vi "convert_then_upload.vi"() -> ()   [LabVIEW 2016]
uses:
  subvi/Data.S3/Data.S3.lvclass
  <userlib>/_OpenG.lib/file/file.llb/File Exists - Scalar__ogtk.vi
  <userlib>/_OpenG.lib/file/file.llb/Build Path - File Names Array__ogtk.vi
panel:
  in  "POPULATE TDMS LIST":bool
  in  "folder with tdms":path
  out "Converting Indicator":bool
  in  "auto upload":bool
  out "of":i32
  out "file #":i32
  out "currently uploading file:":path
  out "errorish":string
  in  "path to aws credentials":path=path "C:/Users/phil/.aws/credentials"
  in  "aws bucket":string="levylab-data"
  out "Uploading Indicator":bool
  out "S3 upload (ms)":u32
  out "generated tdms files (w/ metadata)":path[](array[path])
  in  "UPLOAD CONVERTED":bool
  out "not itx folder":bool[](array[boolean])
  in  "e.g. SA03008N.20190801":path=path "C:/bigdata/PPMS2/SA03008N.20190801"
  in  "Tree":string[](tree)
  in  "CONVERT SELECTED":bool
  in  "OK":bool
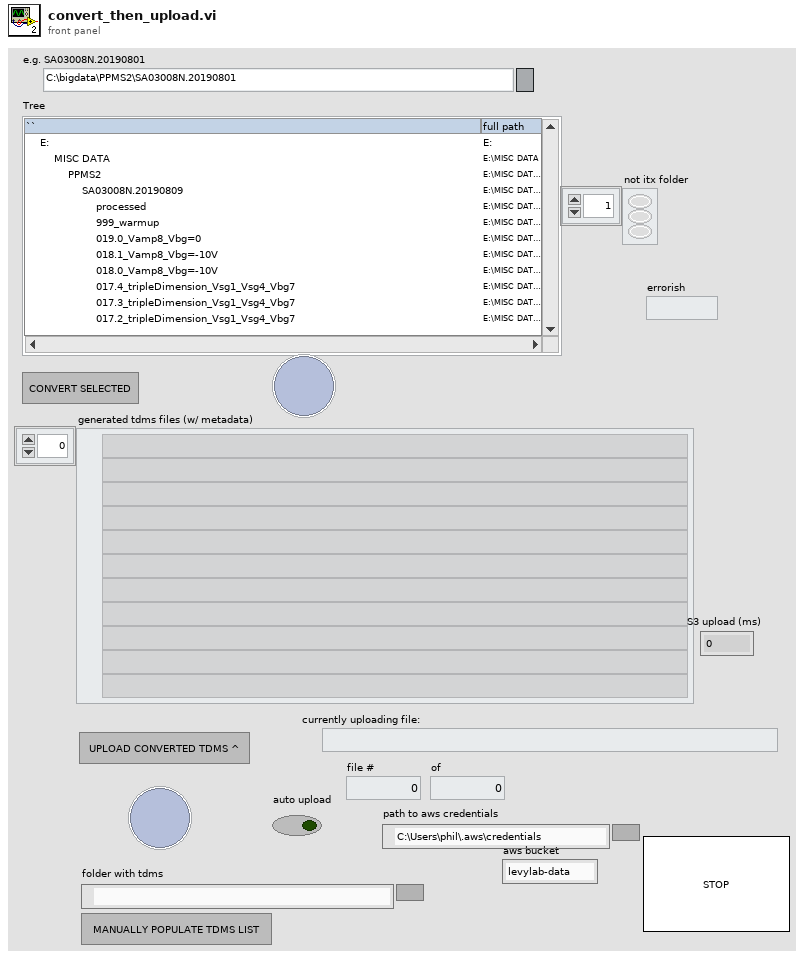
[diagram p1: front panel]
types:
  T1 = enum32{"Invalid", "Standard", "Closed", "Hidden", "Minimized", "Maximized"}
  T2 = enum32{"invalid app kind", "Development System", "Run Time System", "Student Edition", "Embedded LabVIEW", "Evaluation", "Custom"}
  T3 = cluster{"Core":cluster{"Current VI Reference":refnum<vi>, "Close Panel on Exit?":bool}, "Your Boolean data":bool, "e.g. SA03008N.20190801":path, "all expt folders (for tree)":path[], "generated tdms files":path[], "selected folders to convert":path[], "Tree":refnum<vi>, "Data.S3":refnum<class "Data.S3.lvclass">}
  T4 = cluster{"Current VI Reference":refnum<vi>, "Close Panel on Exit?":bool}
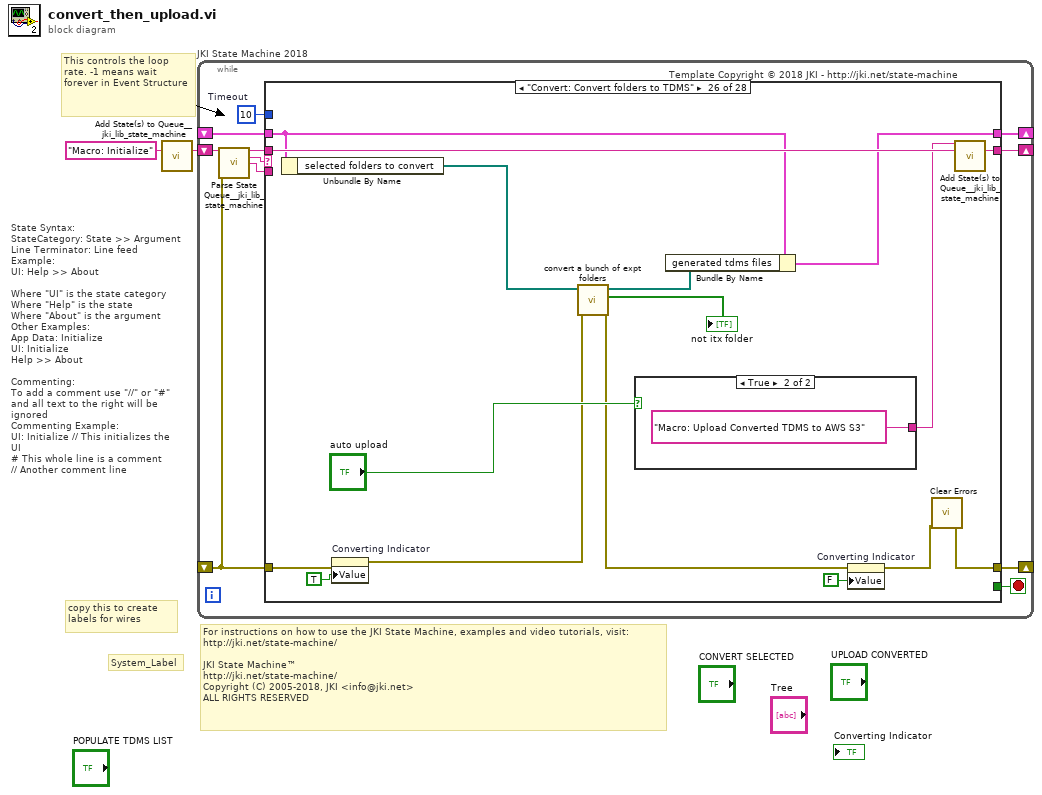
[diagram p0: block diagram]
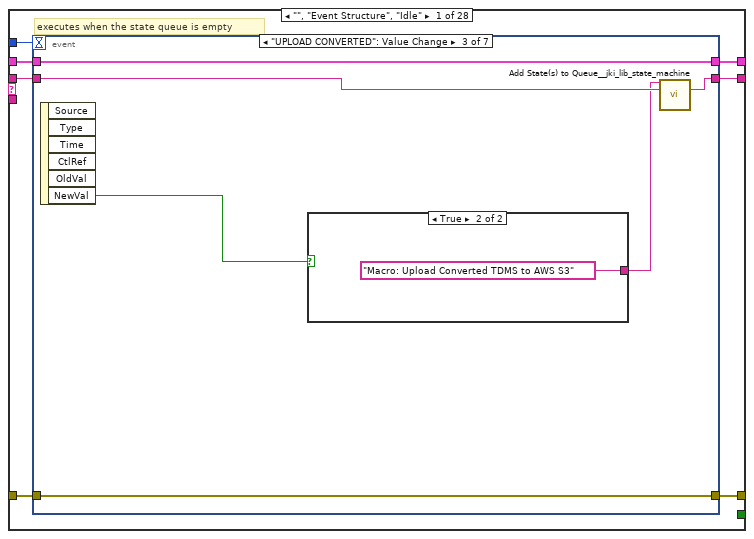
[diagram p2: hidden frame]
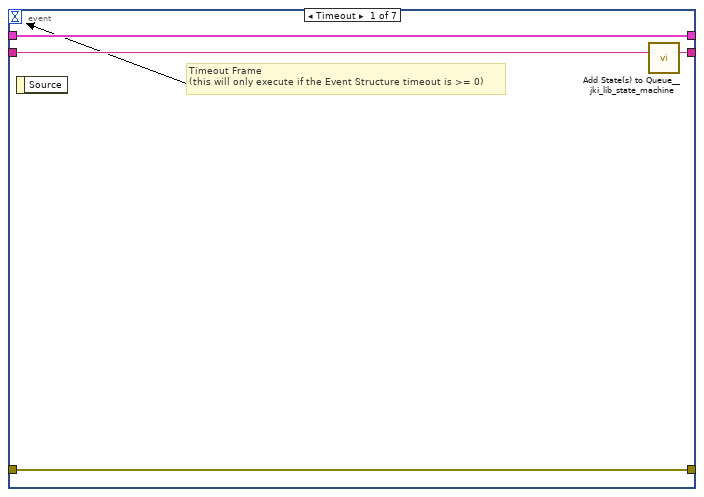
[diagram p3: hidden frame]
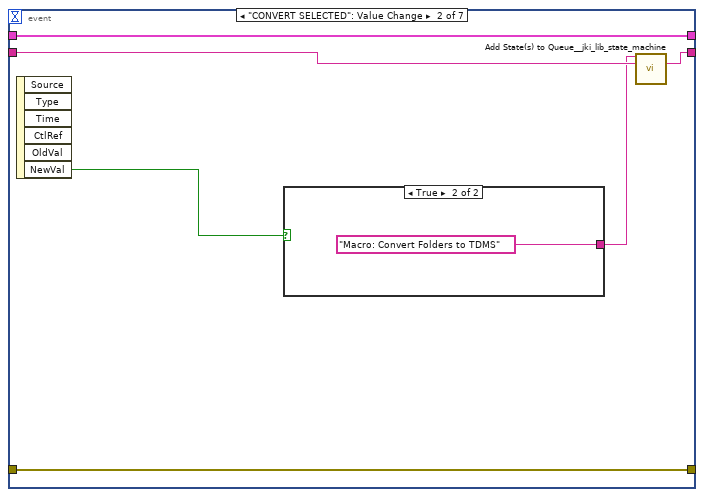
[diagram p4: hidden frame]
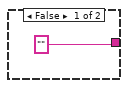
[diagram p5: hidden frame]
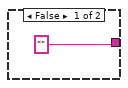
[diagram p6: hidden frame]
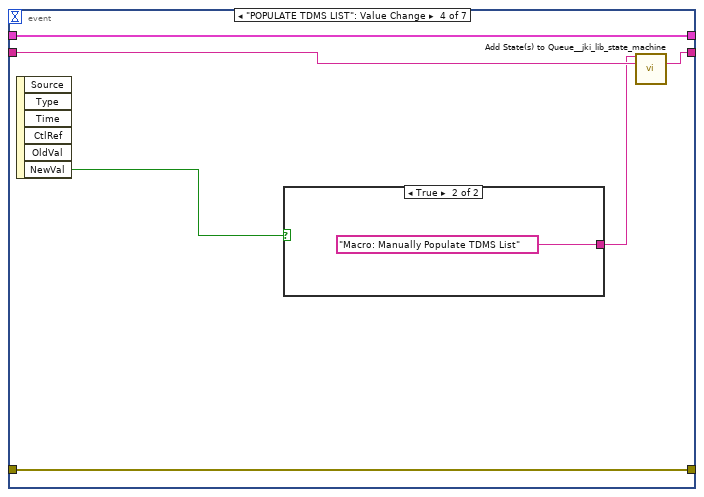
[diagram p7: hidden frame]
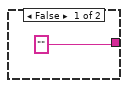
[diagram p8: hidden frame]
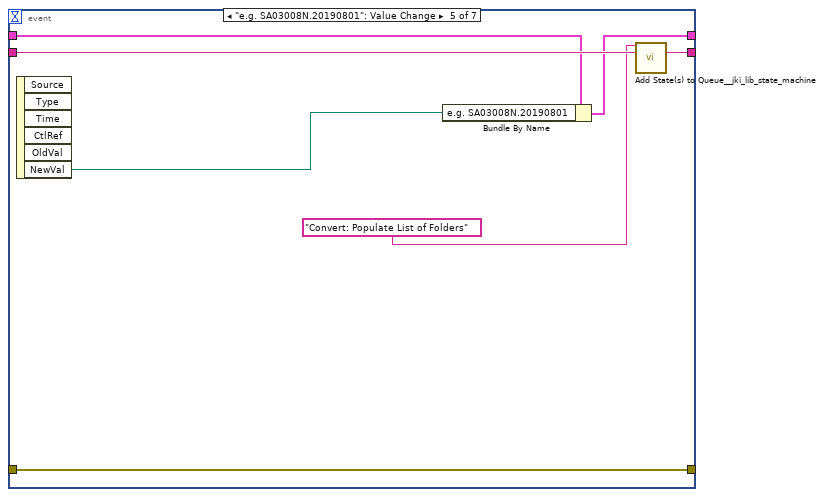
[diagram p9: hidden frame]
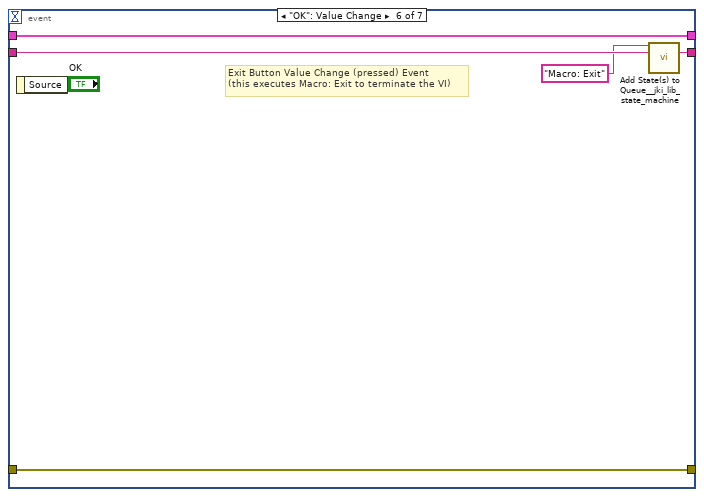
[diagram p10: hidden frame]
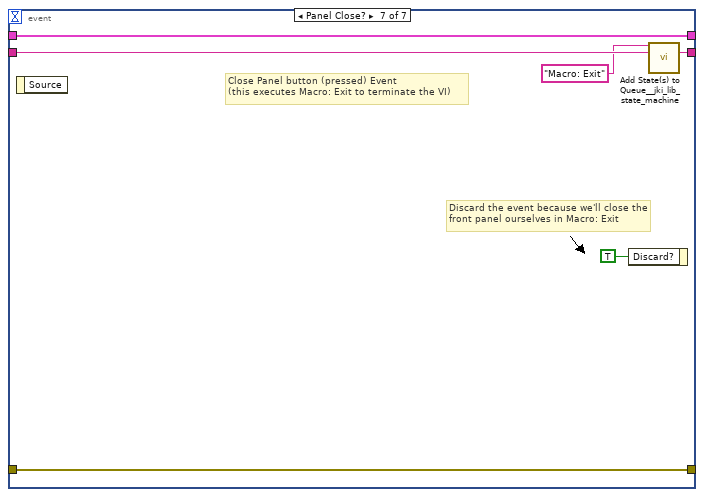
[diagram p11: hidden frame]
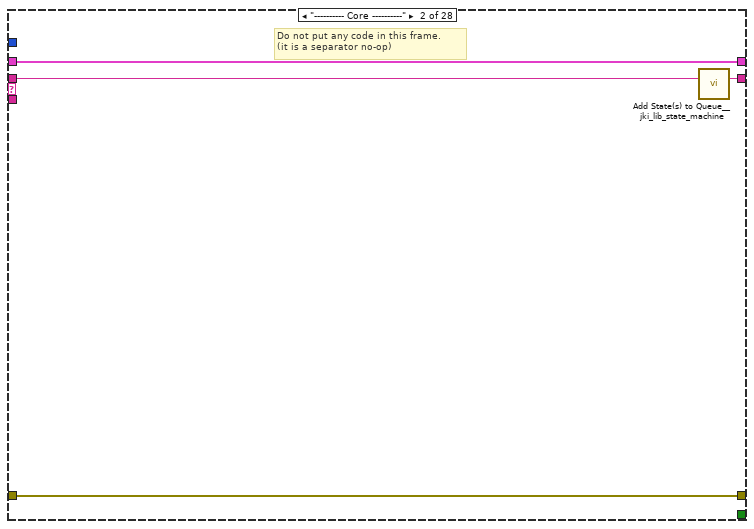
[diagram p12: hidden frame]
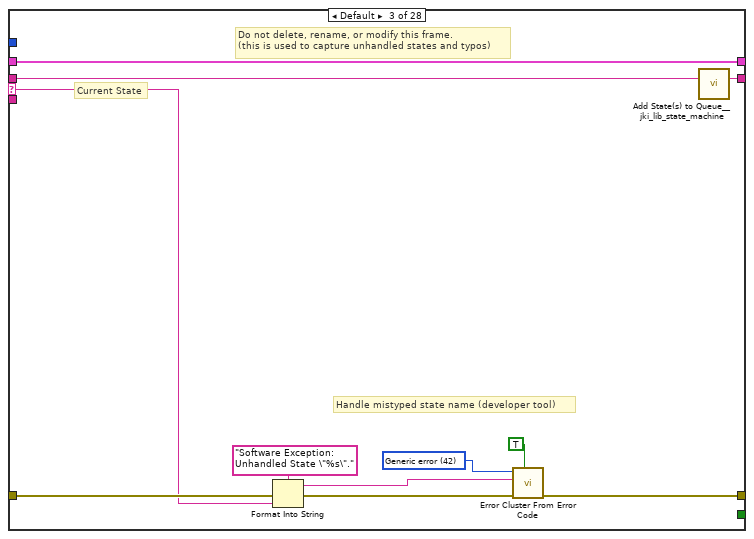
[diagram p13: hidden frame]
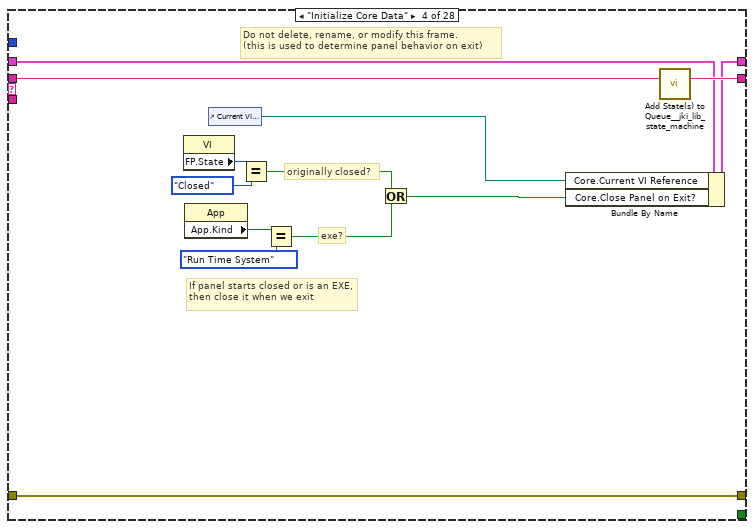
[diagram p14: hidden frame]
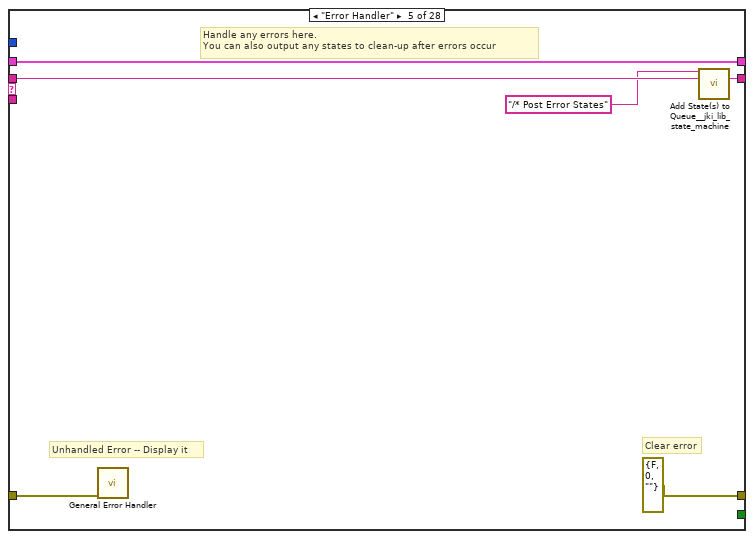
[diagram p15: hidden frame]
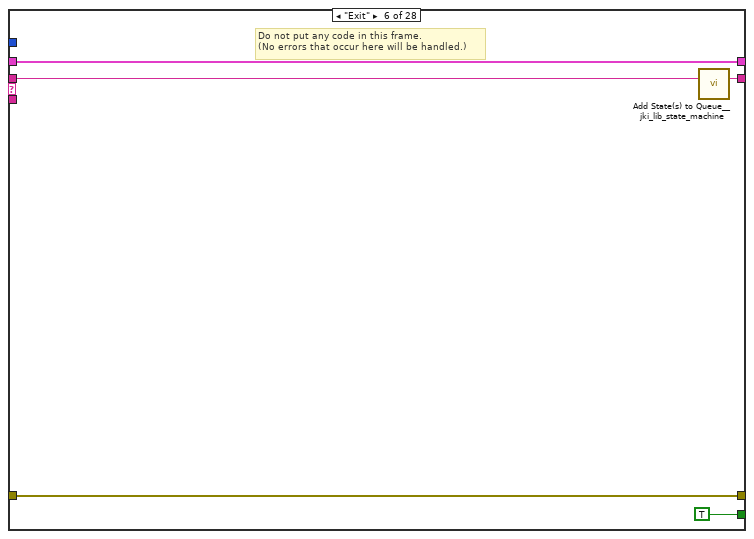
[diagram p16: hidden frame]
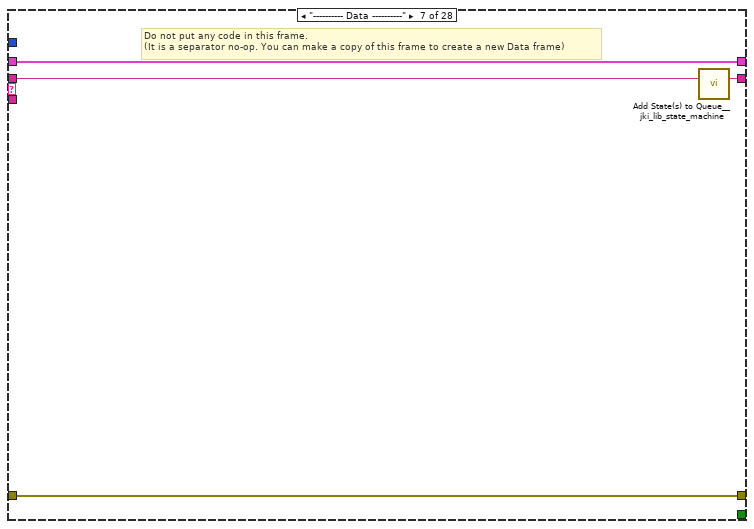
[diagram p17: hidden frame]
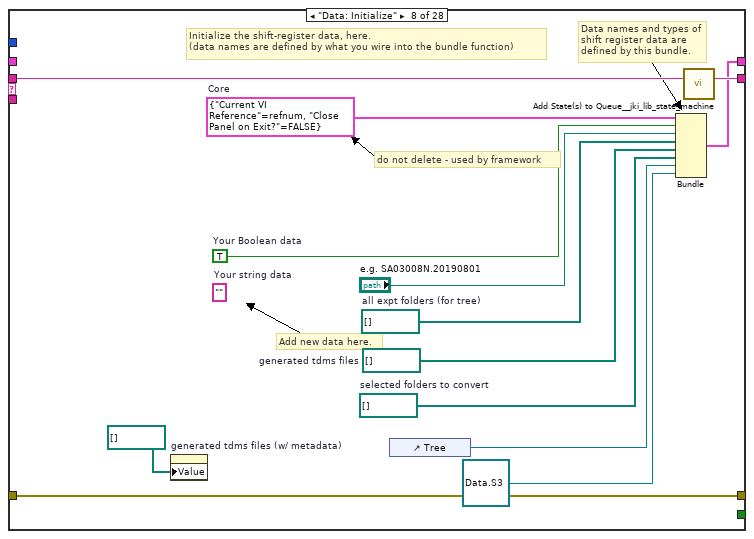
[diagram p18: hidden frame]
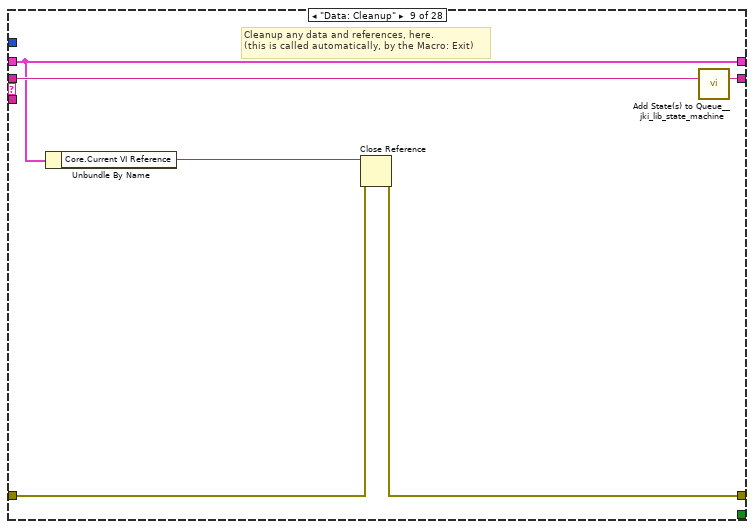
[diagram p19: hidden frame]
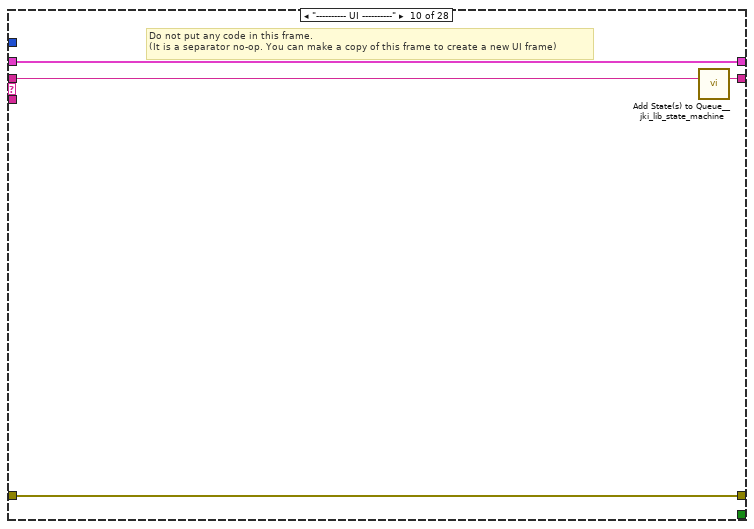
[diagram p20: hidden frame]
diagram:
  # "For instructions on how to use the JKI State Machine, examples and video tutorials, visit:\nhttp://jki.net/state-machine/\n\nJKI State Machine™\nhttp://jki.net/state-machine/\nCopyright (C) 2005-2018, JKI <info@jki.net>\nALL RIGHTS RESERVED"
  # "State Syntax:\nStateCategory: State >> Argument\nLine Terminator: Line feed\nExample:\nUI: Help >> About\n\nWhere \"UI\" is the state category\nWhere \"Help\" is the state\nWhere \"About\" is the argument\nOther Examples:\nApp Data: Initialize\nUI: Initialize\nHelp >> About\n\nCommenting:\nTo add a comment use \"//\" or \"#\" and all text to the right will be ignored\nCommenting Example:\nUI: Initialize // This initializes the UI\n# This whole line is a comment\n// Another comment line"
  # "copy this to create labels for wires"
  # "This controls the loop rate. -1 means wait forever in Event Structure"
  # "System_Label"
  n1 = call <vilib>:"Add State(s) to Queue__jki_lib_state_machine.vi"("State(s) in (\"\")"="Macro: Initialize") -> ("States Out"=w2:string)  [unwired: 14 in]
  n2 = while "JKI State Machine 2018" {
    shift-right: [w6] -> _
    shift-left: _ -> [w5]
    shift-right: [w9] -> _
    shift-left: _ -> [w3]
    shift-right: [w8] -> _
    shift-left: w2 -> [w10]
    stop <- w7 stop-if-true
    w4 = 10  # Timeout
    # "Template Copyright © 2018 JKI - http://jki.net/state-machine"
    n3 = call <vilib>:"Parse State Queue__jki_lib_state_machine.vi"("State Queue"=w10, "Error In (no error)"=w3) -> ("Remaining States"=w12:string, "Current State"=w13:string, "Arguments"=w11:string)  [unwired: 11 in]
    n4 = case shown="\"Convert: Convert folders to TDMS\"" w13 {
      selector: w13 -> [_ _ w71 _ _ _ _ _ _ _ _ _ _ _ _ _ _ _ _ _ _ _ _ _ _ _ _ _]
      tunnel: w12 -> [w20 w70 w75 w94 w100 w105 w109 w122 w128 w132 w136 w142 w153 w222 w227 w232 w237 w242 w252 w256 w275 w323 w331 w345 w359 w375 w382 w391]
      tunnel: w11 -> [_ _ _ _ _ _ _ _ _ _ _ w137 w147 _ _ _ _ _ _ _ _ _ _ _ _ _ _ _]
      tunnel: w5 -> [w18 w67 w73 w87 w97 w103 w106 _ w123 w129 w134 w140 w149 w219 w224 w229 w234 w239 w249 w253 w259 w316 w328 w339 w356 w371 w379 w386]
      tunnel: [w17 w68 w77 w91 errorcluster {"status"=FALSE, "code"=0, "source"=""} ("error out") w102 w107 w119 w124 w130 w133 w138 w150 w220 w225 w230 w235 w240 w250 w254 w273 w313 w329 w332 w351 w360 w380 w388] -> w9
      tunnel: w3 -> [w16 w68 w76 w91 w96 w102 w107 w119 w125 w130 w133 w139 w151 w220 w225 w230 w235 w240 w250 w254 w273 w312 w329 w335 w352 w366 w380 w389]
      tunnel: [w19 w69 w74 w93 w99 w104 w108 w121 w127 w131 w135 w141 w152 w221 w226 w231 w236 w241 w251 w255 w274 w322 w330 w344 w358 w374 w381 w390] -> w8
      tunnel: [_ _ _ _ _ TRUE _ _ _ _ _ _ _ _ _ _ _ _ _ _ _ _ _ _ _ _ _ _] -> w7
      tunnel: [w15 w67 w73 w92 w97 w103 w106 w120 w123 w129 w134 w140 w149 w219 w224 w229 w234 w239 w249 w253 w258 w315 w328 w343 w357 w370 w379 w385] -> w6
      tunnel: w4 -> [w14 _ _ _ _ _ _ _ _ _ _ _ _ _ _ _ _ _ _ _ _ _ _ _ _ _ _ _]
      frame "", "Event Structure", "Idle" {
        # "executes when the state queue is empty"
        n5 = event shown="[2] \"UPLOAD CONVERTED\": Value Change" {
          selector: _ -> [_ _ _ _ _ _ _]
          dyn-events: _ -> [_ _ _ _ _ _ _]
          timeout: w14 -> [_ _ _ _ _ _ _]
          tunnel: w20 -> [w24 w28 w36 w44 w54 w60 w66]
          tunnel: [w23 w29 w37 w45 w55 w59 w65] -> w19
          tunnel: w18 -> [w21 w30 w38 w46 w51 w57 w63]
          tunnel: [w22 w27 w35 w43 w53 w58 w64] -> w17
          tunnel: w16 -> [w22 w27 w35 w43 w53 w58 w64]
          tunnel: [w21 w30 w38 w46 w50 w57 w63] -> w15
          event Timeout {
            # "Timeout Frame\n(this will only execute if the Event Structure timeout is >= 0)"
            n6 = event-data() -> ()  [unwired: 1 in, 1 out]
            n7 = call <vilib>:"Add State(s) to Queue__jki_lib_state_machine.vi"("State(s) in (\"\")"=w24) -> ("States Out"=w23:string)  [unwired: 14 in]
          }
          event "CONVERT SELECTED": Value Change {
            n8 = event-data() -> ("NewVal"=w26:bool)  [unwired: 1 in, 5 out]
            n9 = case shown="True" w26 {
              tunnel: ["" "Macro: Convert Folders to TDMS"] -> w25
              frame False {
              }
              frame True {
              }
            }
            n10 = call <vilib>:"Add State(s) to Queue__jki_lib_state_machine.vi"("State(s) in Front (\"\")"=w25, "State(s) in (\"\")"=w28) -> ("States Out"=w29:string)  [unwired: 13 in]
          }
          event "UPLOAD CONVERTED": Value Change {
            n11 = event-data() -> ("NewVal"=w34:bool)  [unwired: 1 in, 5 out]
            n12 = case shown="True" w34 {
              tunnel: ["" "Macro: Upload Converted TDMS to AWS S3"] -> w33
              frame False {
              }
              frame True {
              }
            }
            n13 = call <vilib>:"Add State(s) to Queue__jki_lib_state_machine.vi"("State(s) in Front (\"\")"=w33, "State(s) in (\"\")"=w36) -> ("States Out"=w37:string)  [unwired: 13 in]
          }
          event "POPULATE TDMS LIST": Value Change {
            n14 = event-data() -> ("NewVal"=w42:bool)  [unwired: 1 in, 5 out]
            n15 = case shown="True" w42 {
              tunnel: ["" "Macro: Manually Populate TDMS List"] -> w41
              frame False {
              }
              frame True {
              }
            }
            n16 = call <vilib>:"Add State(s) to Queue__jki_lib_state_machine.vi"("State(s) in Front (\"\")"=w41, "State(s) in (\"\")"=w44) -> ("States Out"=w45:string)  [unwired: 13 in]
          }
          event "e.g. SA03008N.20190801": Value Change {
            n17 = event-data() -> ("NewVal"=w49:path)  [unwired: 1 in, 5 out]
            n18 = Bundle By Name(cluster=w51, "e.g. SA03008N.20190801"=w49) -> (w50:T3)
            n19 = call <vilib>:"Add State(s) to Queue__jki_lib_state_machine.vi"("State(s) in Front (\"\")"="Convert: Populate List of Folders", "State(s) in (\"\")"=w54) -> ("States Out"=w55:string)  [unwired: 13 in]
          }
          event "OK": Value Change {
            # "Exit Button Value Change (pressed) Event\n(this executes Macro: Exit to terminate the VI)"
            n20 = event-data() -> ()  [unwired: 1 in, 1 out]
            n21 = call <vilib>:"Add State(s) to Queue__jki_lib_state_machine.vi"("State(s) in Front (\"\")"="Macro: Exit", "State(s) in (\"\")"=w60) -> ("States Out"=w59:string)  [unwired: 13 in]
          }
          event Panel Close? {
            # "Discard the event because we'll close the front panel ourselves in Macro: Exit"
            # "Close Panel button (pressed) Event\n(this executes Macro: Exit to terminate the VI)"
            n22 = event-data() -> ()  [unwired: 1 in, 1 out]
            n23 = event-data("Discard?"=TRUE) -> ()  [unwired: 1 in, 1 out]
            n24 = call <vilib>:"Add State(s) to Queue__jki_lib_state_machine.vi"("State(s) in Front (\"\")"="Macro: Exit", "State(s) in (\"\")"=w66) -> ("States Out"=w65:string)  [unwired: 13 in]
          }
        }
      }
      frame "---------- Core ----------" {
        # "Do not put any code in this frame.\n(it is a separator no-op)"
        n25 = call <vilib>:"Add State(s) to Queue__jki_lib_state_machine.vi"("State(s) in (\"\")"=w70) -> ("States Out"=w69:string)  [unwired: 14 in]
      }
      frame Default {
        w80 = 42 items=["No error", "Argument error", "Memory is full", "Out of zone", "End of file", "File already open", "Generic file I/O error", "File not found", "File permission error", "Disk is full", "Duplicate path", "Too many files open", "System feature not enabled", "Resource file not found", "Cannot add resource", "Resource not found", "Image not found", "Image memory error", "Pen does not exist", "Config type invalid", "Config token not found", "Config parse error", "Config memory error", "Bad external code format", "Bad external code offset", "External code not present", "Null window", "Destroy window error", "Null menu", "Print aborted", "Bad print record", "Print driver error", "Windows error during printing", "Memory error during printing", "Print dialog error", "Generic print error", "Invalid device refnum", "Device not found", "Device parameter error", "Device unit error", "Cannot open device", "Device call aborted", "Generic error", "Cancelled by user", "Object ID too low", "Object ID too high", "Object not in heap", "Unknown heap", "Unknown object (invalid DefProc)", "Unknown object (DefProc not in table)", "Message out of range", "Invalid (null) method", "Unknown message", "Manager call not supported", "Bad address", "Network operation in progress", "Network operation timed out", "Connection is busy", "Network attribute not supported", "Network error", "Address in use", "System out of memory", "Connection aborted", "Connection refused", "Not connected", "Already connected", "Connection closed", "Initialization error (interapplication manager)", "Bad occurrence", "Wait on unbound occurrence handler", "Occurrence queue overflow", "Datalog type conflict", "Unused", "Unrecognized type (interapplication manager)", "Memory corrupt", "Failed to make temporary DLL", "Old CIN version", "Drag socket not found", "Failed to load drop-object", "Failed to register OLE object", "Failed to release OLE object", "Format specifier type mismatch", "Unknown format specifier", "Too few format specifiers", "Too many format specifiers", "Scan failed", "Newer CIN version", "Error converting to variant", "Runtime menu error", "Password tampered", "Variant attribute not found", "Incompatible variant data type", "Event data is not available", "Event Store is not present", "Occurrence is not found", "Event Queue is not created", "Event info is not available", "Refnum passed is NULL", "Error retrieving Class GUID", "Error retrieving CoClass GUID", "Error retrieving TypeLib GUID.", "Bad built application magic bytes.", "Specific driver is different from the specific driver associated with the Logical Name.", "There is no session opened to the class driver.", "Max Error", "MAX - Error with config objects", "MAX - Error loading configuration", "MAX - Group not supported"]
        # "Current State"
        # "Do not delete, rename, or modify this frame.\n(this is used to capture unhandled states and typos)"
        # "Handle mistyped state name (developer tool)"
        n26 = Format Into String(format string="Software Exception: Unhandled State \"%s\"." ("message"), error in=w76, w71) -> (resulting string=w79:string, error out=w78:errorcluster)  [unwired: 1 in]
        n27 = call <vilib>:"Error Cluster From Error Code.vi"("show call chain? (False)"=TRUE, "error in (no error)"=w78, "error message (\"\")"=w79, "error code (0)"=w80) -> ("error out"=w77:errorcluster)  [unwired: 5 in]
        n28 = call <vilib>:"Add State(s) to Queue__jki_lib_state_machine.vi"("State(s) in (\"\")"=w75) -> ("States Out"=w74:string)  [unwired: 14 in]
      }
      frame "Initialize Core Data" {
        # "Do not delete, rename, or modify this frame.\n(this is used to determine panel behavior on exit)"
        # "originally closed?"
        # "exe?"
        # "If panel starts closed or is an EXE, then close it when we exit"
        n29 = property class="VI"() -> ("FP.State"=w84:T1)  [unwired: 2 in, 2 out]
        n30 = property class="App"() -> ("App.Kind"=w90:T2)  [unwired: 2 in, 2 out]
        n31 = control-ref of="Current VI Reference"() -> (w85:refnum<vi>)
        n32 = Equal?(x=w84, y=T1."Closed" ("Front Panel Window:State")) -> (x = y?=w82:bool)
        n33 = Equal?(x=w90, y=T2."Run Time System" ("Application:Kind")) -> (x = y?=w88:bool)
        n34 = Or(x=w82, y=w88) -> (x .or. y?=w86:bool)
        n35 = Bundle By Name(cluster=w87, "Core.Current VI Reference"=w85, "Core.Close Panel on Exit?"=w86) -> (w92:T3)
        n36 = call <vilib>:"Add State(s) to Queue__jki_lib_state_machine.vi"("State(s) in (\"\")"=w94) -> ("States Out"=w93:string)  [unwired: 14 in]
      }
      frame "Error Handler" {
        # "Unhandled Error -- Display it"
        # "Handle any errors here.\nYou can also output any states to clean-up after errors occur"
        # "Clear error"
        n37 = call <vilib>:"General Error Handler.vi"("error in (no error)"=w96) -> ()  [unwired: 10 in, 5 out]
        n38 = call <vilib>:"Add State(s) to Queue__jki_lib_state_machine.vi"("State(s) in Front (\"\")"="/* Post Error States", "State(s) in (\"\")"=w100) -> ("States Out"=w99:string)  [unwired: 13 in]
      }
      frame "Exit" {
        # "Do not put any code in this frame.\n(No errors that occur here will be handled.)"
        n39 = call <vilib>:"Add State(s) to Queue__jki_lib_state_machine.vi"("State(s) in (\"\")"=w105) -> ("States Out"=w104:string)  [unwired: 14 in]
      }
      frame "---------- Data ----------" {
        # "Do not put any code in this frame.\n(It is a separator no-op. You can make a copy of this frame to create a new Data frame)"
        n40 = call <vilib>:"Add State(s) to Queue__jki_lib_state_machine.vi"("State(s) in (\"\")"=w109) -> ("States Out"=w108:string)  [unwired: 14 in]
      }
      frame "Data: Initialize" {
        w114 = path[] []  # selected folders to convert
        w115 = path[] []  # generated tdms files
        w116 = path[] []  # all expt folders (for tree)
        w117 = T4 {"Current VI Reference"=refnum, "Close Panel on Exit?"=FALSE}  # Core
        w118 = TRUE  # Your Boolean data
        (unwired) ""  # Your string data
        # "do not delete - used by framework"
        # "Add new data here."
        # "Data names and types of shift register data are defined by this bundle."
        # "Initialize the shift-register data, here.\n(data names are defined by what you wire into the bundle function)"
        n41 = property on="generated tdms files (w/ metadata)" class="Arr (strict)"("Value"=path[] [] ("converted folders")) -> ()  [unwired: 2 in, 2 out]
        n42 = control-ref of="Tree"() -> (w112:refnum<vi>)
        n43 = Bundle("Core"=w117, "Your Boolean data"=w118, "e.g. SA03008N.20190801"="e.g. SA03008N.20190801", "all expt folders (for tree)"=w116, "generated tdms files"=w115, "selected folders to convert"=w114, "Tree"=w112, "Data.S3"=refnum<class "Data.S3.lvclass"> refnum) -> (w120:T3)  [unwired: 1 in]
        n44 = call <vilib>:"Add State(s) to Queue__jki_lib_state_machine.vi"("State(s) in (\"\")"=w122) -> ("States Out"=w121:string)  [unwired: 14 in]
      }
      frame "Data: Cleanup" {
        # "Cleanup any data and references, here.\n(this is called automatically, by the Macro: Exit)"
        n45 = Unbundle By Name(w123) -> ("Core.Current VI Reference"=w126:refnum<vi>)
        n46 = Close Reference(reference=w126, error in (no error)=w125) -> (error out=w124:errorcluster)
        n47 = call <vilib>:"Add State(s) to Queue__jki_lib_state_machine.vi"("State(s) in (\"\")"=w128) -> ("States Out"=w127:string)  [unwired: 14 in]
      }
      frame "---------- UI ----------" {
        # "Do not put any code in this frame.\n(It is a separator no-op. You can make a copy of this frame to create a new UI frame)"
        n48 = call <vilib>:"Add State(s) to Queue__jki_lib_state_machine.vi"("State(s) in (\"\")"=w132) -> ("States Out"=w131:string)  [unwired: 14 in]
      }
      frame "UI: Initialize" {
        # "Initialize the User Interface, here.\n(this is called automatically, by the Macro: Init)"
        n49 = call <vilib>:"Add State(s) to Queue__jki_lib_state_machine.vi"("State(s) in (\"\")"=w136) -> ("States Out"=w135:string)  [unwired: 14 in]
      }
      frame "UI: Cursor Set" {
        # "Argument"
        # "Set and Unset Cursor Busy.\n(Usage: \"UI: Cursor Set >> Busy|Idle\")"
        n50 = case shown="\"Idle\", Default" w137 {
          tunnel: w139 -> [w144 w146]
          tunnel: [w143 w145] -> w138
          frame "Idle", Default {
            n51 = call <vilib>:"Unset Busy.vi"("error in (no error)"=w144) -> ("error out"=w143:errorcluster)  [unwired: 10 in]
          }
          frame "Busy" {
            n52 = call <vilib>:"Set Busy.vi"("error in (no error)"=w146) -> ("error out"=w145:errorcluster)  [unwired: 9 in, 1 out]
          }
        }
        n53 = call <vilib>:"Add State(s) to Queue__jki_lib_state_machine.vi"("State(s) in (\"\")"=w142) -> ("States Out"=w141:string)  [unwired: 14 in]
      }
      frame "UI: Front Panel State" {
        # "Argument"
        # "Set Front Panel Open or Closed\n(Usage: \"UI: Front Panel State >> Open|Close\")"
        n54 = Unbundle By Name(w149) -> ("Core.Current VI Reference"=w148:refnum<vi>)
        n55 = case shown="\"Minimize\", \"Minimized\"" w147 {
          tunnel: w151 -> [w159 w174 w185 w198 w211]
          tunnel: [w161 w175 w187 w200 w213] -> w150
          tunnel: w148 -> [w160 w172 w186 w199 w212]
          frame "Open", "Standard", Default {
            w154 = T1."Standard" ("State")
            n56 = property class="VI"(reference=w160, error in=w159) -> (reference out=w157:refnum<vi>, error out=w158:errorcluster, "FP.State"=w156:T1)
            n57 = Not Equal?(x=w156, y=w154) -> (x != y?=w155:bool)
            n58 = case shown="True" w155 {
              tunnel: [w165 w167] -> w161
              tunnel: w158 -> [w164 w167]
              tunnel: w157 -> [w163 _]
              tunnel: w154 -> [w162 _]
              frame True {
                n59 = invoke class="VI" method="FP.Open"(reference=w163, error in=w164, "Activate"=TRUE, "State"=w162) -> (error out=w165:errorcluster)  [unwired: 1 in, 4 out]
              }
              frame False {
              }
            }
          }
          frame "Close", "Closed" {
            n60 = property class="VI"(reference=w172, error in=w174) -> (reference out=w171:refnum<vi>, error out=w173:errorcluster, "FP.State"=w169:T1)
            n61 = Not Equal?(x=w169, y=T1."Closed" ("Front Panel Window:State")) -> (x != y?=w168:bool)
            n62 = case shown="True" w168 {
              tunnel: [w176 w179] -> w175
              tunnel: w173 -> [w176 w178]
              tunnel: w171 -> [_ w177]
              frame False {
              }
              frame True {
                n63 = invoke class="VI" method="FP.Close"(reference=w177, error in=w178) -> (error out=w179:errorcluster)  [unwired: 1 in, 2 out]
              }
            }
          }
          frame "Hidden", "Hide" {
            w180 = T1."Hidden" ("State")
            n64 = property class="VI"(reference=w186, error in=w185) -> (reference out=w183:refnum<vi>, error out=w184:errorcluster, "FP.State"=w182:T1)
            n65 = Not Equal?(x=w182, y=w180) -> (x != y?=w181:bool)
            n66 = case shown="True" w181 {
              tunnel: [w191 w192] -> w187
              tunnel: w184 -> [w190 w192]
              tunnel: w183 -> [w189 _]
              tunnel: w180 -> [w188 _]
              frame True {
                n67 = invoke class="VI" method="FP.Open"(reference=w189, error in=w190, "State"=w188) -> (error out=w191:errorcluster)  [unwired: 2 in, 4 out]
              }
              frame False {
              }
            }
          }
          frame "Minimize", "Minimized" {
            w193 = T1."Minimized" ("State")
            n68 = property class="VI"(reference=w199, error in=w198) -> (reference out=w196:refnum<vi>, error out=w197:errorcluster, "FP.State"=w195:T1)
            n69 = Not Equal?(x=w195, y=w193) -> (x != y?=w194:bool)
            n70 = case shown="True" w194 {
              tunnel: [w204 w205] -> w200
              tunnel: w197 -> [w203 w205]
              tunnel: w196 -> [w202 _]
              tunnel: w193 -> [w201 _]
              frame True {
                n71 = invoke class="VI" method="FP.Open"(reference=w202, error in=w203, "State"=w201) -> (error out=w204:errorcluster)  [unwired: 2 in, 4 out]
              }
              frame False {
              }
            }
          }
          frame "Maximize", "Maximized" {
            w206 = T1."Maximized" ("State")
            n72 = property class="VI"(reference=w212, error in=w211) -> (reference out=w209:refnum<vi>, error out=w210:errorcluster, "FP.State"=w208:T1)
            n73 = Not Equal?(x=w208, y=w206) -> (x != y?=w207:bool)
            n74 = case shown="True" w207 {
              tunnel: [w217 w218] -> w213
              tunnel: w210 -> [w216 w218]
              tunnel: w209 -> [w215 _]
              tunnel: w206 -> [w214 _]
              frame True {
                n75 = invoke class="VI" method="FP.Open"(reference=w215, error in=w216, "State"=w214) -> (error out=w217:errorcluster)  [unwired: 2 in, 4 out]
              }
              frame False {
              }
            }
          }
        }
        n76 = call <vilib>:"Add State(s) to Queue__jki_lib_state_machine.vi"("State(s) in (\"\")"=w153) -> ("States Out"=w152:string)  [unwired: 14 in]
      }
      frame "---------- Macro ----------" {
        # "Do not put any code in this frame.\n(It is a separator no-op. You can make a copy of this frame to create a new Macro frame)"
        n77 = call <vilib>:"Add State(s) to Queue__jki_lib_state_machine.vi"("State(s) in (\"\")"=w222) -> ("States Out"=w221:string)  [unwired: 14 in]
      }
      frame "Macro: Initialize" {
        w223 = "Data: Initialize\nInitialize Core Data\nUI: Initialize\nUI: Front Panel State >> Open\nConvert: Populate List of Folders\nAWS: Initialize"  # Data: Initialize Initialize Core Data UI: Initialize UI: Front Panel State >> Open Convert: Populate List of Folders AWS: Initialize
        # "Initialization Macro\n(This is called once, when the VI starts)"
        n78 = call <vilib>:"Add State(s) to Queue__jki_lib_state_machine.vi"("State(s) in Front (\"\")"=w223, "State(s) in (\"\")"=w227) -> ("States Out"=w226:string)  [unwired: 13 in]
      }
      frame "Macro: Convert Folders to TDMS" {
        # "Initialization Macro\n(This is called once, when the VI starts)"
        n79 = call <vilib>:"Add State(s) to Queue__jki_lib_state_machine.vi"("State(s) in Front (\"\")"="Convert: Obtain Selected Folders\nConvert: Convert folders to TDMS\nConvert: Update TDMS List", "State(s) in (\"\")"=w232) -> ("States Out"=w231:string)  [unwired: 13 in]
      }
      frame "Macro: Upload Converted TDMS to AWS S3" {
        # "Initialization Macro\n(This is called once, when the VI starts)"
        n80 = call <vilib>:"Add State(s) to Queue__jki_lib_state_machine.vi"("State(s) in Front (\"\")"="AWS: Upload Converted TDMS", "State(s) in (\"\")"=w237) -> ("States Out"=w236:string)  [unwired: 13 in]
      }
      frame "Macro: Manually Populate TDMS List" {
        # "Initialization Macro\n(This is called once, when the VI starts)"
        n81 = call <vilib>:"Add State(s) to Queue__jki_lib_state_machine.vi"("State(s) in Front (\"\")"="Convert: Populate TDMS List from Folder\nConvert: Update TDMS List", "State(s) in (\"\")"=w242) -> ("States Out"=w241:string)  [unwired: 13 in]
      }
      frame "Macro: Exit" {
        # "Exit Macro\n(This is called once, when the VI exits)"
        n82 = Unbundle By Name(w249) -> ("Core.Close Panel on Exit?"=w248:bool)
        n83 = Select(t="UI: Front Panel State >> Close", s=w248, f="") -> (s? t:f=w245:string)
        n84 = call <vilib>:"Add State(s) to Queue__jki_lib_state_machine.vi"("State(s) in (\"\")"=w245, "State(s) at Back (\"\")"="Data: Cleanup\nExit") -> ("States Out"=w243:string)  [unwired: 13 in]
        n85 = call <vilib>:"Add State(s) to Queue__jki_lib_state_machine.vi"("State(s) in Front (\"\")"=w243, "State(s) in (\"\")"=w252) -> ("States Out"=w251:string)  [unwired: 13 in]
      }
      frame "---------- AWS ----------" {
        # "Template Separator\n(You can make a copy of, or modify, this frame)"
        n86 = Unbundle By Name(w253) -> ()  [unwired: 1 out]
        n87 = call <vilib>:"Add State(s) to Queue__jki_lib_state_machine.vi"("State(s) in (\"\")"=w256) -> ("States Out"=w255:string)  [unwired: 14 in]
      }
      frame "AWS: Upload Converted TDMS" {
        # "Template Separator\n(You can make a copy of, or modify, this frame)"
        # "Your code here.\n(You can make a copy of, or modify, this frame)"
        n88 = control-ref of="Uploading Indicator"() -> (w269:refnum<vi>)
        n89 = property on="Property Node" class="Bool (strict)"(reference=w269, "Value"=TRUE ("Downloading Indicator")) -> (reference out=w268:refnum<vi>, error out=w267:errorcluster)  [unwired: 1 in]
        n90 = Unbundle By Name(w259) -> ("generated tdms files"=w257:path[], "Data.S3"=w272:refnum<class "Data.S3.lvclass">)
        n91 = call <userlib>:"Tick Count (ms)__ogtk.vi"("error in (no error)"=w267) -> ("error out"=w266:errorcluster, "millisecond timer value"=w262:u32)  [unwired: 9 in]
        n92 = for {
          tunnel: w272 -> [w293]
          tunnel: [w285] -> w260
          shift-right: [w278] -> w265
          shift-left: w266 -> [w286]
          tunnel: w257 -> [w283] mode=indexing
          tunnel: w257 -> [w280]
          i -> [w282]
          w288 = "/"
          # "PPMS2"
          # "reformat name"
          # "SA030.."
          # "031_.."
          # "#TODO: put these values in the\nstate wire..."
          n93 = Array Size(array=w280) -> (size(s)=→"of":i32)
          n94 = Strip Path(path=w283) -> (stripped path=w299:path, name=w298:string)
          n95 = Strip Path(path=w299) -> (stripped path=w291:path, name=w296:string)
          n96 = call "replace_bad_aws_characters.vi"("error in (no error)"=w286, "name"=w298) -> ("error out"=w294:errorcluster, "result string"=w297:string)  [unwired: 8 in]
          n97 = Strip Path(path=w291) -> (name=w290:string)  [unwired: 1 out]
          n98 = call "replace_bad_aws_characters.vi"("error in (no error)"=w294, "name"=w296) -> ("error out"=w289:errorcluster, "result string"=w295:string)  [unwired: 8 in]
          n99 = call-poly <userlib>:"File Exists__ogtk.vi"("file path"=w283) -> ("exists"=w284:bool)  [unwired: 6 in, 1 out]
          n100 = call "replace_bad_aws_characters.vi"("error in (no error)"=w289, "name"=w290) -> ("error out"=w277:errorcluster, "result string"=w287:string)  [unwired: 8 in]
          n101 = Concatenate Strings(w288, w287, w288, w295, w288, w297) -> (w292:string)
          n102 = call <vilib>:"Clear Errors.vi"("error in (no error)"=w277) -> ("error out"=w276:errorcluster)  [unwired: 5 in, 1 out]
          n103 = case shown="False" w284 {
            tunnel: w283 -> [w304 w306]
            tunnel: w292 -> [_ w311]
            tunnel: w276 -> [w300 w310]
            tunnel: [w300 w309] -> w279
            tunnel: w293 -> [w305 w308]
            tunnel: [w305 w307] -> w285
            frame False {
              n104 = Path To String(path=w304) -> (string=w302:string)
              n105 = Concatenate Strings("bad", w302) -> (→"errorish":string)
            }
            frame True {
              n106 = call "Upload File.vi"("error in (no error)"=w310, "Object Path (including file name)"=w311, "file to upload"=w306, "Data.S3"=w308) -> ("error out"=w309:errorcluster, "Data.S3"=w307:refnum<class "Data.S3.lvclass">)  [unwired: 6 in]
            }
          }
          n107 = call <vilib>:"Clear Errors.vi"("error in (no error)"=w279) -> ("error out"=w278:errorcluster)  [unwired: 5 in, 1 out]
          "currently uploading file:" <- w283
          "file #" <- w282
        }
        n108 = call <userlib>:"Tick Count (ms)__ogtk.vi"("error in (no error)"=w265) -> ("error out"=w264:errorcluster, "millisecond timer value"=w263:u32)  [unwired: 9 in]
        n109 = Subtract(x=w263, y=w262) -> (x-y=→"S3 upload (ms)":u32)
        n110 = property on="Property Node" class="Bool (strict)"(reference=w268, error in=w264, "Value"=FALSE ("Downloading Indicator")) -> ()  [unwired: 2 out]
        n111 = Bundle By Name(cluster=w259, "Data.S3"=w260) -> (w258:T3)
        n112 = call <vilib>:"Add State(s) to Queue__jki_lib_state_machine.vi"("State(s) in (\"\")"=w275) -> ("States Out"=w274:string)  [unwired: 14 in]
      }
      frame "AWS: Initialize" {
        # "need to somehow set credentials and bucket"
        # "Your code here.\n(You can make a copy of, or modify, this frame)"
        n113 = Unbundle By Name(w316) -> ("Data.S3"=w321:refnum<class "Data.S3.lvclass">)
        n114 = call-poly <userlib>:"File Exists__ogtk.vi"("file path"="path to aws credentials") -> ("exists"=w317:bool)  [unwired: 6 in, 1 out]
        n115 = case shown="True" w317 {
          tunnel: w321 -> [w324 w327]
          tunnel: [w324 w326] -> w319
          tunnel: "path to aws credentials" -> [_ w325]
          frame False {
          }
          frame True {
            n116 = call "Read Credentials from File.vi"("path to aws credentials"=w325, "Data.S3"=w327) -> ("Data.S3 out"=w326:refnum<class "Data.S3.lvclass">)  [unwired: 8 in, 1 out]
          }
        }
        n117 = call "Set Bucket.vi"("error in (no error)"=w312, "Bucket name"="aws bucket", "Data.S3"=w319) -> ("error out"=w313:errorcluster, "Data.S3"=w314:refnum<class "Data.S3.lvclass">)  [unwired: 7 in]
        n118 = Bundle By Name(cluster=w316, "Data.S3"=w314) -> (w315:T3)
        n119 = call <vilib>:"Add State(s) to Queue__jki_lib_state_machine.vi"("State(s) in (\"\")"=w323) -> ("States Out"=w322:string)  [unwired: 14 in]
      }
      frame "---------- Convert ----------" {
        # "Template Separator\n(You can make a copy of, or modify, this frame)"
        n120 = call <vilib>:"Add State(s) to Queue__jki_lib_state_machine.vi"("State(s) in (\"\")"=w331) -> ("States Out"=w330:string)  [unwired: 14 in]
      }
      frame "Convert: Populate List of Folders" {
        # "Template Separator\n(You can make a copy of, or modify, this frame)"
        n121 = Unbundle By Name(w339) -> ("e.g. SA03008N.20190801"=w338:path, "Tree"=w336:refnum<vi>)
        n122 = List Folder(path=w338) -> (path out=w342:path, folder names=w341:string[])  [unwired: 3 in, 2 out]
        n123 = invoke class="Tree (strict)" method="Edit Tree Items.Delete"(reference=w336, error in=w335) -> (reference out=w337:refnum<vi>, error out=w334:errorcluster)  [unwired: 3 in, 3 out]
        n124 = call-poly <userlib>:"Build Path__ogtk.vi"("name or relative path"=w341, "base path"=w342) -> ("appended path"=w340:path[])
        n125 = for {
          tunnel: w334 -> [w350]
          tunnel: [w349] -> w333
          tunnel: w340 -> [w347] mode=indexing
          tunnel: w337 -> [w346]
          n126 = Path To String(path=w347) -> (string=w348:string)
          n127 = call "recursively populate local multi-tree ctl.vi"("error in (no error)"=w350, "multi-selectable tree ctl ref"=w346, "Object path"=w348) -> ("error out"=w349:errorcluster)  [unwired: 7 in, 1 out]
        }
        n128 = call <vilib>:"Clear Errors.vi"("error in (no error)"=w333) -> ("error out"=w332:errorcluster)  [unwired: 5 in, 1 out]
        n129 = Bundle By Name(cluster=w339, "all expt folders (for tree)"=w340) -> (w343:T3)
        n130 = call <vilib>:"Add State(s) to Queue__jki_lib_state_machine.vi"("State(s) in (\"\")"=w345) -> ("States Out"=w344:string)  [unwired: 14 in]
      }
      frame "Convert: Obtain Selected Folders" {
        # "Template Separator\n(You can make a copy of, or modify, this frame)"
        n131 = Unbundle By Name(w356) -> ("Tree"=w355:refnum<vi>)
        n132 = property class="Tree (strict)"(reference=w355, error in=w352) -> (error out=w351:errorcluster, "Value"=w354:string[])  [unwired: 1 out]
        n133 = String To Path(string=w354) -> (path=w353:path[])
        n134 = Bundle By Name(cluster=w356, "selected folders to convert"=w353) -> (w357:T3)
        n135 = call <vilib>:"Add State(s) to Queue__jki_lib_state_machine.vi"("State(s) in (\"\")"=w359) -> ("States Out"=w358:string)  [unwired: 14 in]
      }
      frame "Convert: Convert folders to TDMS" {
        n136 = Unbundle By Name(w371) -> ("selected folders to convert"=w373:path[])
        n137 = property on="Converting Indicator" class="Bool (strict)"(error in=w366, "Value"=TRUE ("Converting Indicator")) -> (error out=w364:errorcluster)  [unwired: 1 in, 1 out]
        n138 = call "convert a bunch of expt folders.vi"("error in (no error)"=w364, "Array of expt folders"=w373) -> ("error out"=w365:errorcluster, "not itx folder"=→"not itx folder":bool[], "generated tdms files (w/ metadata)"=w372:path[])  [unwired: 7 in]
        n139 = case shown="True" "auto upload" {
          tunnel: ["" "Macro: Upload Converted TDMS to AWS S3"] -> w367
          frame False {
          }
          frame True {
          }
        }
        n140 = Bundle By Name(cluster=w371, "generated tdms files"=w372) -> (w370:T3)
        n141 = property on="Converting Indicator" class="Bool (strict)"(error in=w365, "Value"=FALSE ("Converting Indicator")) -> (error out=w361:errorcluster)  [unwired: 1 in, 1 out]
        n142 = call <vilib>:"Clear Errors.vi"("error in (no error)"=w361) -> ("error out"=w360:errorcluster)  [unwired: 5 in, 1 out]
        n143 = call <vilib>:"Add State(s) to Queue__jki_lib_state_machine.vi"("State(s) in Front (\"\")"=w367, "State(s) in (\"\")"=w375) -> ("States Out"=w374:string)  [unwired: 13 in]
      }
      frame "Convert: Update TDMS List" {
        n144 = Unbundle By Name(w379) -> ("generated tdms files"=→"generated tdms files (w/ metadata)":path[])
        n145 = call <vilib>:"Add State(s) to Queue__jki_lib_state_machine.vi"("State(s) in (\"\")"=w382) -> ("States Out"=w381:string)  [unwired: 14 in]
      }
      frame "Convert: Populate TDMS List from Folder" {
        n146 = call <vilib>:"Recursive File List.vi"("pattern"="*.tdms", "error in (no error)"=w389, "Folder Path"="folder with tdms") -> ("error out"=w388:errorcluster, "All Files in Dir"=w383:path[])  [unwired: 4 in, 3 out]
        n147 = Bundle By Name(cluster=w386, "generated tdms files"=w383) -> (w385:T3)
        n148 = call <vilib>:"Add State(s) to Queue__jki_lib_state_machine.vi"("State(s) in (\"\")"=w391) -> ("States Out"=w390:string)  [unwired: 14 in]
      }
    }
  }
